vi "UpdateErrorAcq.vi"(8 "error in (no error)":errorcluster, 11 "Acquisition in":refnum<class "Acquisition.lvclass">) -> (0 "error out":errorcluster, 1 "STOP":bool, 3 "Acquisition out":refnum<class "Acquisition.lvclass">)   [LabVIEW 2014, in "Acquisition.lvclass"]
uses:
  Acquisition.lvclass
  Acquisition.lvclass/Acquisition.ctl
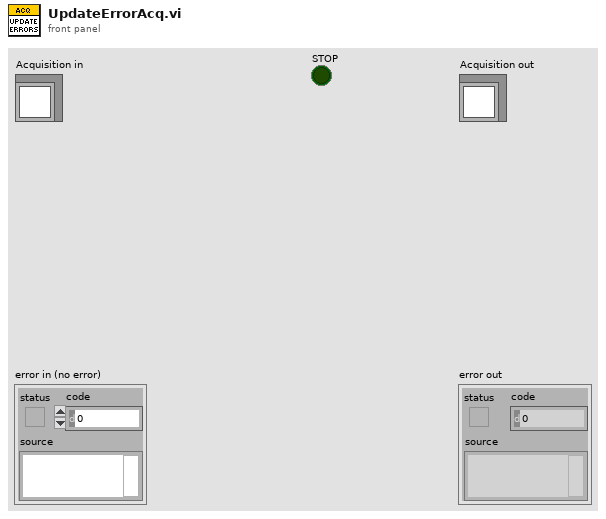
[diagram p1: front panel]
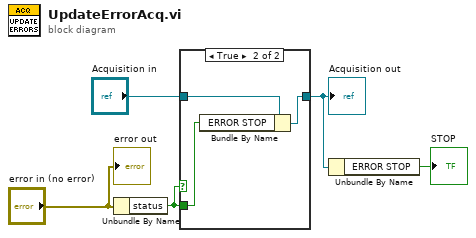
[diagram p0: block diagram]
diagram:
  n1 = Unbundle By Name("error in (no error)") -> ("status"=w3:bool)
  n2 = case shown="True" w3 {
    tunnel: "Acquisition in" -> [w6 w9]
    tunnel: [w6 w8] -> w2
    tunnel: w3 -> [_ w7]
    frame False {
    }
    frame True {
      n3 = Bundle By Name(cluster=w9, "ERROR STOP"=w7) -> (w8:refnum<class "Acquisition.lvclass">)
    }
  }
  "Acquisition out" <- w2
  n4 = Unbundle By Name(w2) -> ("ERROR STOP"=→"STOP":bool)
  "error out" <- "error in (no error)"
